vi "Add Big Noise.vi"(11 "channel 1":T2) -> (3 "channel 2":T1)   [LabVIEW 2019]
doc: "Given a value coming in on a channel, disturb that value by a significant amount of noise."
uses:
  <extravilib>/ChannelInstances/Stream-i32/)Channel.ctl
  <extravilib>/ChannelInstances/Stream-dbl/)Channel.ctl
  <extravilib>/ChannelInstances/Stream-i32/Read With Abort.vi
  <extravilib>/ChannelInstances/Stream-dbl/Write With Abort.vi
  <extravilib>/ChannelInstances/Stream-i32/EndpointRead.vi
  <extravilib>/ChannelInstances/Stream-dbl/Endpoint.vi
  <extravilib>/ChannelInstances/Stream-i32/)Channel.vi
  <resource>/ChannelSupport/_ChannelSupport/WaitIfNeeded.vi
  <extravilib>/ChannelInstances/Stream-dbl/)Channel.vi
  <extravilib>/ChannelInstances/Stream-i32.lvlib
  <extravilib>/ChannelInstances/Stream-dbl.lvlib
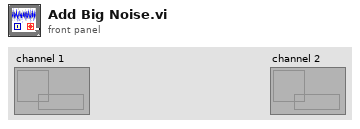
[diagram p1: front panel]
types:
  T1 = typedef "Stream-dbl.lvlib/)Channel.ctl" = refnum<queue>
  T2 = typedef "Stream-i32.lvlib/)Channel.ctl" = refnum<queue>
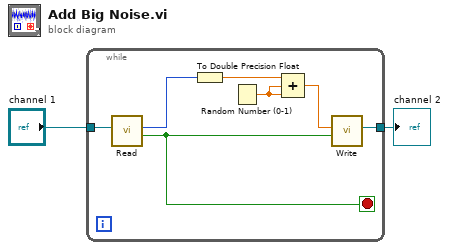
[diagram p0: block diagram]
diagram:
  n1 = while {
    tunnel: [w4] -> w1
    tunnel: "channel 1" -> [w7]
    stop <- w5 stop-if-true
    n2 = call <extravilib>:"Read.vi"("channel"=w7) -> ("last element?"=w5:bool, "element"=w6:i32)  [unwired: 6 in, 3 out]
    n3 = To Double Precision Float(number=w6) -> (double precision float=w3:dbl)
    n4 = Random Number (0-1)() -> (number: 0 to 1=w8:dbl)
    n5 = Compound Arithmetic op=ADD(w3, w8, w8) -> (w9:dbl)
    n6 = call <extravilib>:"Write.vi"("last element? (F)"=w5, "element"=w9) -> ("channel"=w4:T1)  [unwired: 7 in, 2 out]
  }
  "channel 2" <- w1
